vi "Clusters.vi"(8 "error in (no error)":errorcluster, 11 "System Config in":refnum<class "System Config.lvclass">) -> (0 "error out":errorcluster, 2 "Clusters":refnum<class "Cluster Config.lvclass">[](array[class]), 3 "System Config out":refnum<class "System Config.lvclass">)   [LabVIEW 2020, in "VolatusConfig.lvlib" / "System Config.lvclass"]
uses:
  System Config.lvclass
  System Config.lvclass/System Config.ctl
  VolatusConfigElement/VolatusConfigElement.lvclass
  VolatusConfig.lvlib
  Meta Type.ctl
  Cluster/Cluster Config.lvclass
  C:/dev/lv20CE/relink/lv-volatus/VolatusConfig/VolatusConfigElement/VolatusConfigElement.lvclass
  C:/dev/lv20CE/relink/lv-volatus/VolatusConfig/System/System Config.lvclass
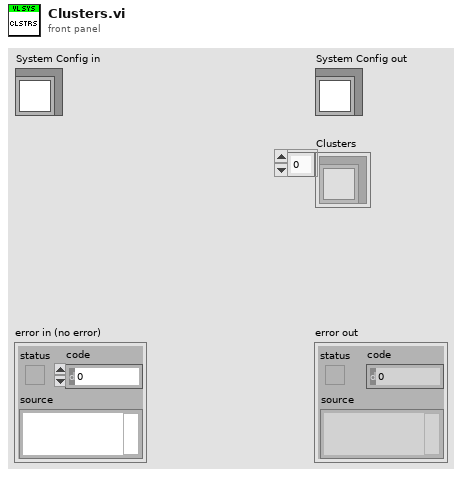
[diagram p1: front panel]
types:
  T1 = typedef "VolatusConfig.lvlib/Meta Type.ctl" = enum16{"UNKNOWN", "VL_System", "VL_Cluster", "VL_Node", "VL_Task", "VL_Group", "VL_Channel", "VL_Task_List", "VL_Scaling", "VL_Sensor", "VL_Sensor_List", "VL_Scale"}
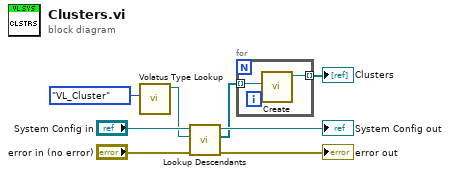
[diagram p0: block diagram]
diagram:
  n1 = call "Volatus Type Lookup.vi"("Meta Type"=Meta_Type."VL_Cluster") -> ("Config Lookup out"=w3:refnum<class "Config Lookup.lvclass">)  [unwired: 9 in, 1 out]
  n2 = call "Lookup Descendants.vi"("error in (no error)"="error in (no error)", "Lookup"=w3, "VolatusConfigElement in"="System Config in") -> ("error out"=→"error out":errorcluster, "Descendants"=w2:refnum<class "Config Element.lvclass">[], "VolatusConfigElement out"=→"System Config out":refnum<class "System Config.lvclass">)  [unwired: 6 in]
  n3 = for {
    tunnel: w2 -> [w10] mode=indexing
    tunnel: [w9] -> w1 mode=indexing
    n4 = call "Create.vi"("Element"=w10) -> ("Cluster out"=w9:refnum<class "Cluster Config.lvclass">)  [unwired: 9 in, 1 out]
  }
  "Clusters" <- w1
